vi "Error 5010.vi"(8 "error in (no error)":errorcluster, 10 "RPC Method Name":string) -> (0 "error out":errorcluster)   [LabVIEW 2019, in "gRPC Template Creation Utility.lvlib"]
uses:
  gRPC Template Creation Utility.lvlib
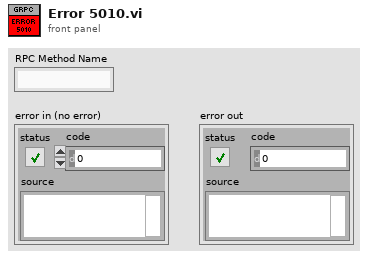
[diagram p1: front panel]
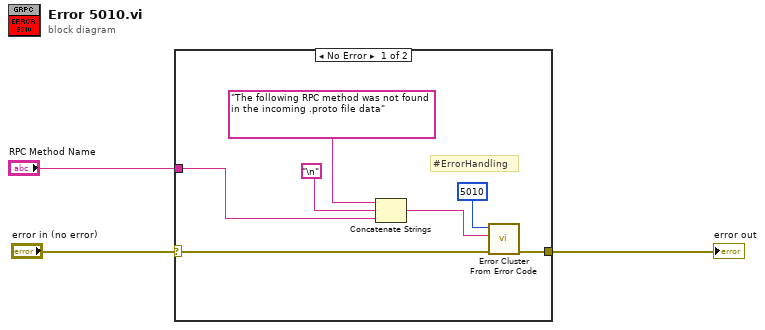
[diagram p0: block diagram]
diagram:
  n1 = case shown="No Error" "error in (no error)" {
    selector: "error in (no error)" -> [w4 w11]
    tunnel: [w10 w11] -> w3
    tunnel: "RPC Method Name" -> [w8 _]
    frame No Error {
      # "#ErrorHandling"
      n2 = Concatenate Strings("The following RPC method was not found in the incoming .proto file data" ("error message (\"\")"), "\n", w8) -> (w9:string)
      n3 = call <vilib>:"Error Cluster From Error Code.vi"("error in (no error)"=w4, "error message (\"\")"=w9, "error code (0)"=5010) -> ("error out"=w10:errorcluster)  [unwired: 6 in]
    }
    frame Error {
    }
  }
  "error out" <- w3
